vi "Recall Van Der Pauw Results.vi"() -> (2 "Van Der Pauw Results":T1)   [LabVIEW 2016, in "Hall Effect Library.lvlib"]
uses:
  Hall Effect Library.lvlib
  Private/Global Variables/Hall Effect Data.vi
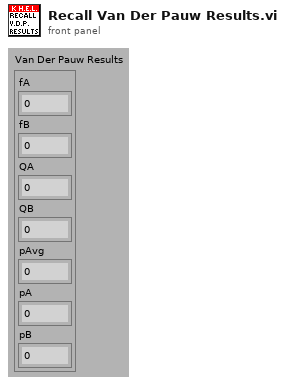
[diagram p1: front panel]
types:
  T1 = cluster{"fA":dbl, "fB":dbl, "QA":dbl, "QB":dbl, "pAvg":dbl, "pA":dbl, "pB":dbl}
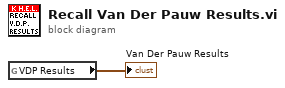
[diagram p0: block diagram]
diagram:
  n1 = global read "Hall Effect Data.vi" "VDP Results"() -> (→"Van Der Pauw Results":T1)
